vi "GenerateFrequencyTable.vi"(6 "amplitude [V]":dbl=0.1, 7 "Oktave/Dekade":enum16{"Dekade", "Oktave"}(ring), 8 "error in":errorcluster, 9 "EndFrequenz":dbl=10000.0, 10 "StartFrequenz":dbl=10.0, 11 "Messungen/Intervall":i32=10) -> (0 "error out":errorcluster, 2 "Frequenzen":dbl[](array[numeric]), 3 "Frequency List":T1(array[cluster]))   [LabVIEW 2012]
panel:
  out "Anzahl der Frequenzen":i32
  out "Intervallgrenzen":T2(array[cluster])
  # "Dieses Vi erzeugt eine Tabelle mit Frequenzen und der zugehörigen Amplitude"
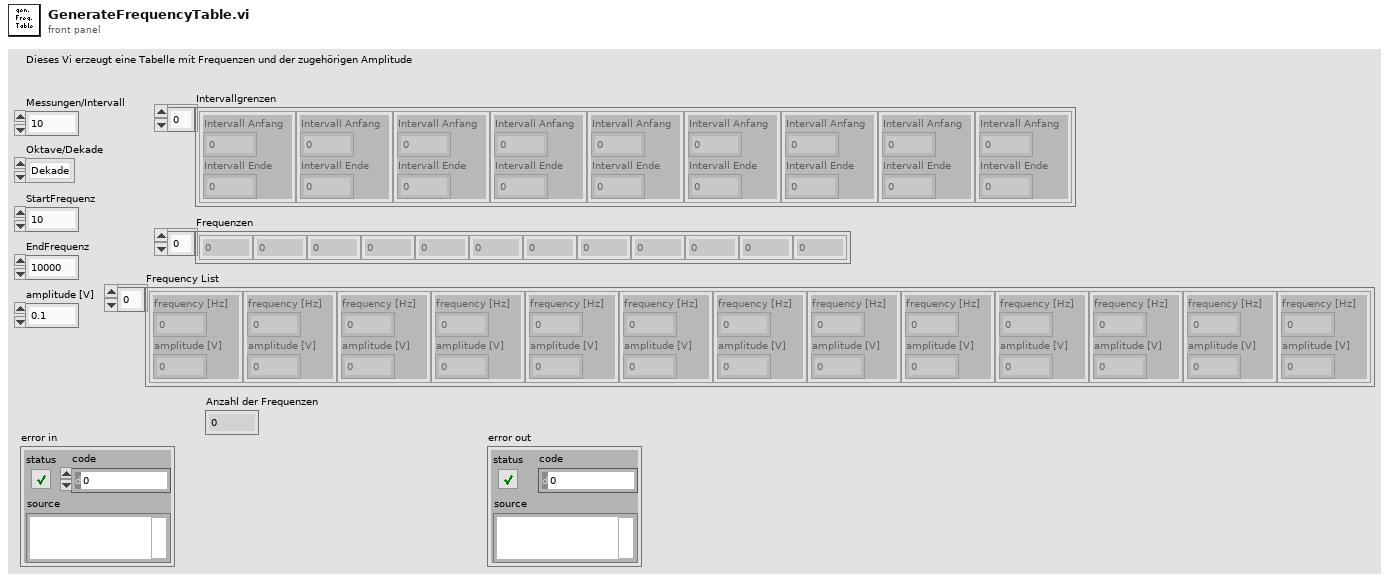
[diagram p1: front panel]
types:
  T1 = cluster{"frequency [Hz]":dbl, "amplitude [V]":dbl}[]
  T2 = cluster{"Intervall Anfang":dbl, "Intervall Ende":dbl}[]
  T3 = cluster{"Intervall Anfang":dbl, "Intervall Ende":dbl}
  T4 = cluster{"frequency [Hz]":dbl, "amplitude [V]":dbl}
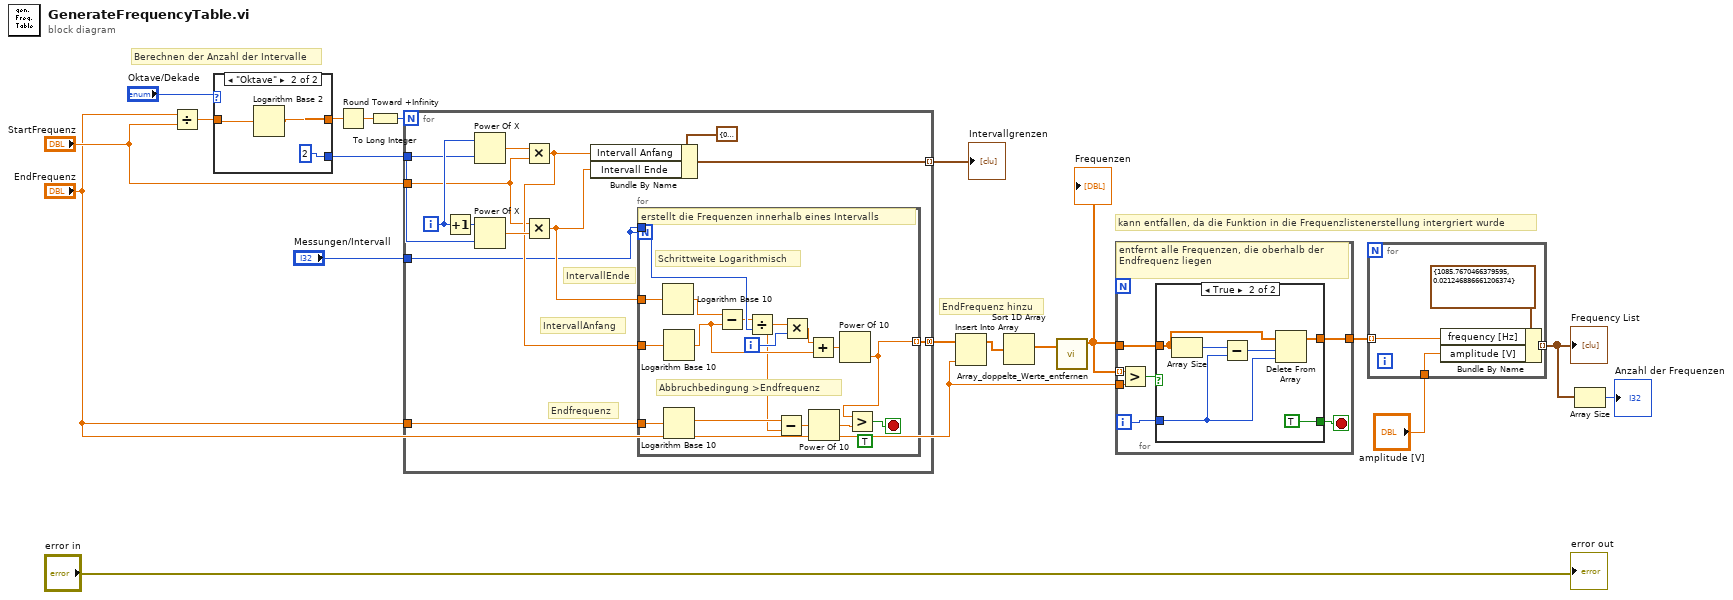
[diagram p0: block diagram]
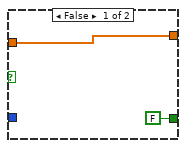
[diagram p2: hidden frame]
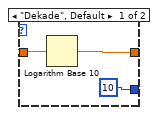
[diagram p3: hidden frame]
diagram:
  # "Berechnen der Anzahl der Intervalle"
  # "kann entfallen, da die Funktion in die Frequenzlistenerstellung intergriert wurde"
  # "EndFrequenz hinzu"
  n1 = Divide(x="EndFrequenz", y="StartFrequenz") -> (x/y=w18:dbl)
  n2 = case shown="\"Oktave\"" "Oktave/Dekade" {
    tunnel: w18 -> [w22 w25]
    tunnel: [w21 w24] -> w17
    tunnel: [10 2] -> w16
    frame "Dekade", Default {
      n3 = Logarithm Base 10(1:w22) -> (0:w21:dbl)
    }
    frame "Oktave" {
      n4 = Logarithm Base 2(1:w25) -> (0:w24:dbl)
    }
  }
  n5 = Round Toward +Infinity(x=w17) -> (ceil(x): smallest int >= x=w14:dbl)
  n6 = To Long Integer(number=w14) -> (32bit integer=w13:i32)
  n7 = for {
    N: w13 -> [_]
    tunnel: w16 -> [w32]
    tunnel: "StartFrequenz" -> [w27]
    tunnel: [w35] -> w15 mode=indexing
    tunnel: "Messungen/Intervall" -> [w29]
    tunnel: [w28] -> w10 mode=concatenating
    tunnel: "EndFrequenz" -> [w26]
    i -> [w34]
    # "Endfrequenz"
    # "IntervallAnfang"
    # "IntervallEnde"
    n8 = Increment(x=w34) -> (x+1=w33:i32)
    n9 = Power Of X(1:w32, 2:w34) -> (0:w37:dbl)
    n10 = Power Of X(1:w32, 2:w33) -> (0:w38:dbl)
    n11 = Multiply(x=w37, y=w27) -> (x*y=w31:dbl)
    n12 = Multiply(x=w27, y=w38) -> (x*y=w30:dbl)
    n13 = Bundle By Name(cluster=T3 {"Intervall Anfang"=0.0, "Intervall Ende"=0.0} ("input cluster"), "Intervall Anfang"=w31, "Intervall Ende"=w30) -> (w35:T3)
    n14 = for {
      N: w29 -> [_]
      tunnel: w29 -> [w54]
      tunnel: w31 -> [w53]
      tunnel: w30 -> [w52]
      tunnel: [w47] -> w28 mode=indexing
      tunnel: w26 -> [w40]
      i -> [w51]
      stop <- w39 stop-if-true
      (unwired) TRUE ("stop")
      # "Abbruchbedingung >Endfrequenz"
      # "Schrittweite Logarithmisch"
      # "erstellt die Frequenzen innerhalb eines Intervalls"
      n15 = Logarithm Base 10(1:w52) -> (0:w45:dbl)
      n16 = Logarithm Base 10(1:w53) -> (0:w49:dbl)
      n17 = Logarithm Base 10(1:w40) -> (0:w42:dbl)
      n18 = Subtract(x=w45, y=w49) -> (x-y=w44:dbl)
      n19 = Divide(x=w44, y=w54) -> (x/y=w41:dbl)
      n20 = Subtract(x=w42, y=w41) -> (x-y=w43:dbl)
      n21 = Multiply(x=w41, y=w51) -> (x*y=w50:dbl)
      n22 = Add(x=w50, y=w49) -> (x+y=w48:dbl)
      n23 = Power Of 10(x=w43) -> (10^x=w46:dbl)
      n24 = Power Of 10(x=w48) -> (10^x=w47:dbl)
      n25 = Greater?(x=w47, y=w46) -> (0:w39:bool)
    }
  }
  "Intervallgrenzen" <- w15
  n26 = Insert Into Array(array=w10, new element="EndFrequenz") -> (w8:dbl[])  [unwired: 1 in]
  n27 = Sort 1D Array(array=w8) -> (sorted array=w7:dbl[])
  n28 = call "Array_doppelte_Werte_entfernen.vi"("Array"=w7) -> ("Array ohne Duplikate"=w6:dbl[])  [unwired: 9 in, 1 out]
  "Frequenzen" <- w6
  n29 = for {
    tunnel: w6 -> [w61] mode=indexing
    tunnel: "EndFrequenz" -> [w60]
    tunnel: w6 -> [w57]
    tunnel: [w56] -> w5
    i -> [w58]
    stop <- w55 stop-if-true
    # "entfernt alle Frequenzen, die oberhalb der Endfrequenz liegen"
    n30 = Greater?(x=w61, y=w60) -> (0:w59:bool)
    n31 = case shown="True" w59 {
      tunnel: w58 -> [_ w65]
      tunnel: w57 -> [w63 w69]
      tunnel: [w63 w68] -> w56
      tunnel: [FALSE TRUE] -> w55
      frame False {
      }
      frame True {
        n32 = Array Size(array=w69) -> (size(s)=w64:i32)
        n33 = Subtract(x=w64, y=w65) -> (x-y=w66:i32)
        n34 = Delete From Array(array=w69, length=w66, index=w65) -> (array with subset deleted=w68:dbl[])  [unwired: 1 out]
      }
    }
  }
  n35 = for {
    tunnel: w5 -> [w72] mode=indexing
    tunnel: [w71] -> w3 mode=indexing
    tunnel: "amplitude [V]" -> [w70]
    n36 = Bundle By Name(cluster=T4 {"frequency [Hz]"=1085.7670466379595, "amplitude [V]"=0.021246886661206374} ("tone settings 2"), "frequency [Hz]"=w72, "amplitude [V]"=w70) -> (w71:T4)
  }
  "Frequency List" <- w3
  n37 = Array Size(array=w3) -> (size(s)=→"Anzahl der Frequenzen":i32)
  "error out" <- "error in"
